vi "Fgen Channel UI.vi"() -> ()   [LabVIEW 2025, in "Fgen.lvlib" / "Fgen Channel.lvclass"]
doc: "Copyright 2017 National Instruments Corporation\n\nLicensed under the Apache License, Version 2.0 (the \"License\"); you may not use this file except in compliance with the License. You may obtain a copy of the License at http://www.apache.org/licenses/LICENSE-2.0\nUnless required by applicable law or agreed to in writing, software distributed under the License is distributed on an \"AS IS\" BASIS, WITHOUT WARRANTIES OR CONDITIONS OF ANY KIND, either express or implied. See the License for the specific language governing permissions and limitations under the License."
uses:
  Fgen Channel.lvclass
  Users/Public/Documents/Sandia National Labs/TSS Plugin/CEF.lvlibp/Node/NodeRef.ctl
  Users/Public/Documents/Sandia National Labs/TSS Plugin/CEF.lvlibp/Node/CEF_Node.lvclass
  Users/Public/Documents/Sandia National Labs/TSS Plugin/CEF.lvlibp/Node/mainQref.ctl
  Users/Public/Documents/Sandia National Labs/TSS Plugin/CEF.lvlibp/Node/UserEventRef.ctl
  Users/Public/Documents/Sandia National Labs/TSS Plugin/Abstract Engine.lvlibp/Plugin/Abstract/Channel configuration/Default Channel.ctl
  Fgen Channel configuration/Fgen Channel Setting.ctl
  Fgen Instrument/Fgen Instrument.lvclass
  Fgen Channel.lvclass/Fgen Channel.ctl
  Fgen Channel configuration/Fgen Channel configuration.lvclass/Fgen Channel configuration.ctl
  Fgen configuration/Fgen configuration.lvclass
  Fgen Channel configuration/Read Fgen Channel.vi
  Fgen Channel configuration/Write Fgen Channel.vi
  <vilib>/Utility/error.llb/Trim Whitespace One-Sided.vi
  Fgen Channel configuration/Fgen Channel configuration.lvclass
  Users/Public/Documents/Sandia National Labs/TSS Plugin/Abstract Engine.lvlibp/Plugin/Abstract/Channel configuration/Read Channel Setting.vi
  Users/Public/Documents/Sandia National Labs/TSS Plugin/CEF.lvlibp/Node/ReadParent.vi
  Users/Public/Documents/Sandia National Labs/TSS Plugin/Abstract Engine.lvlibp/Plugin/Abstract/Instrument configuration/Read Instrument Setting.vi
  Users/Public/Documents/Sandia National Labs/TSS Plugin/Abstract Engine.lvlibp/Plugin/Abstract/Channel configuration/Write Channel Setting.vi
  Users/Public/Documents/Sandia National Labs/TSS Plugin/CEF.lvlibp/serializable configuration/CEF_serializable configuration.lvclass
  Users/Public/Documents/Sandia National Labs/TSS Plugin/Abstract Engine.lvlibp/Plugin/Abstract/Channel configuration/Channel configuration.lvclass
panel:
  in  "Fgen Channel":cluster{"Default":T1, "Setting":T2}={"Default"={"Address"="None", "SW Alias"="Fgen Channel0", "Enabled"=TRUE, "Type"="Fgen Channel", "Description"="* Type = Channel Class"}, "Setting"={"Trgger Type"="Immediate", "Duty Cycle"=0.0, "Amplitude"=0.0, "Frequency"=0.0, "Output Shape"="Sine Wave", "Phase"=0.0}} {"Setting"."Duty Cycle" format="%#_6f"; "Setting"."Frequency" format="%#_6p"; "Setting"."Amplitude" format="%#_6f"}
  in  "user event":T3
  in  "main queue":T4
  in  "node ref":T5
  # "Standard only"
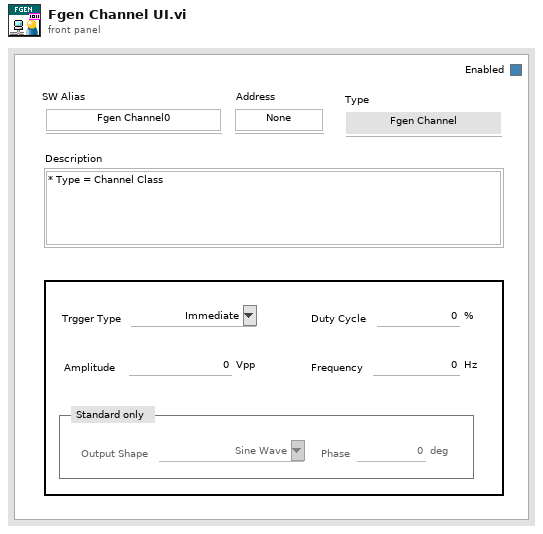
[diagram p1: front panel]
types:
  T1 = typedef "Abstract Engine.lvlibp/Channel configuration.lvclass/Default Channel.ctl" = cluster{"Address":string, "SW Alias":string, "Enabled":bool, "Type":string, "Description":string}
  T2 = typedef "Fgen.lvlib/Fgen Channel configuration.lvclass/Fgen Channel Setting.ctl" = cluster{"Trgger Type":string, "Duty Cycle":dbl, "Amplitude":dbl, "Frequency":dbl, "Output Shape":string, "Phase":dbl}
  T3 = typedef "CEF.lvlibp/CEF_Node.lvclass/UserEventRef.ctl" = refnum<user-event>
  T4 = typedef "CEF.lvlibp/CEF_Node.lvclass/mainQref.ctl" = refnum<queue>
  T5 = typedef "CEF.lvlibp/CEF_Node.lvclass/NodeRef.ctl" = refnum<data-value>
  T6 = typedef "Abstract Engine.lvlibp/Instrument configuration.lvclass/Default Instrument.ctl" = cluster{"Type":string, "Address":string, "SW Alias":string, "Description":string, "Enabled":bool}
  T7 = enum8{"Enabled", "Disabled", "Disabled and Grayed Out"}
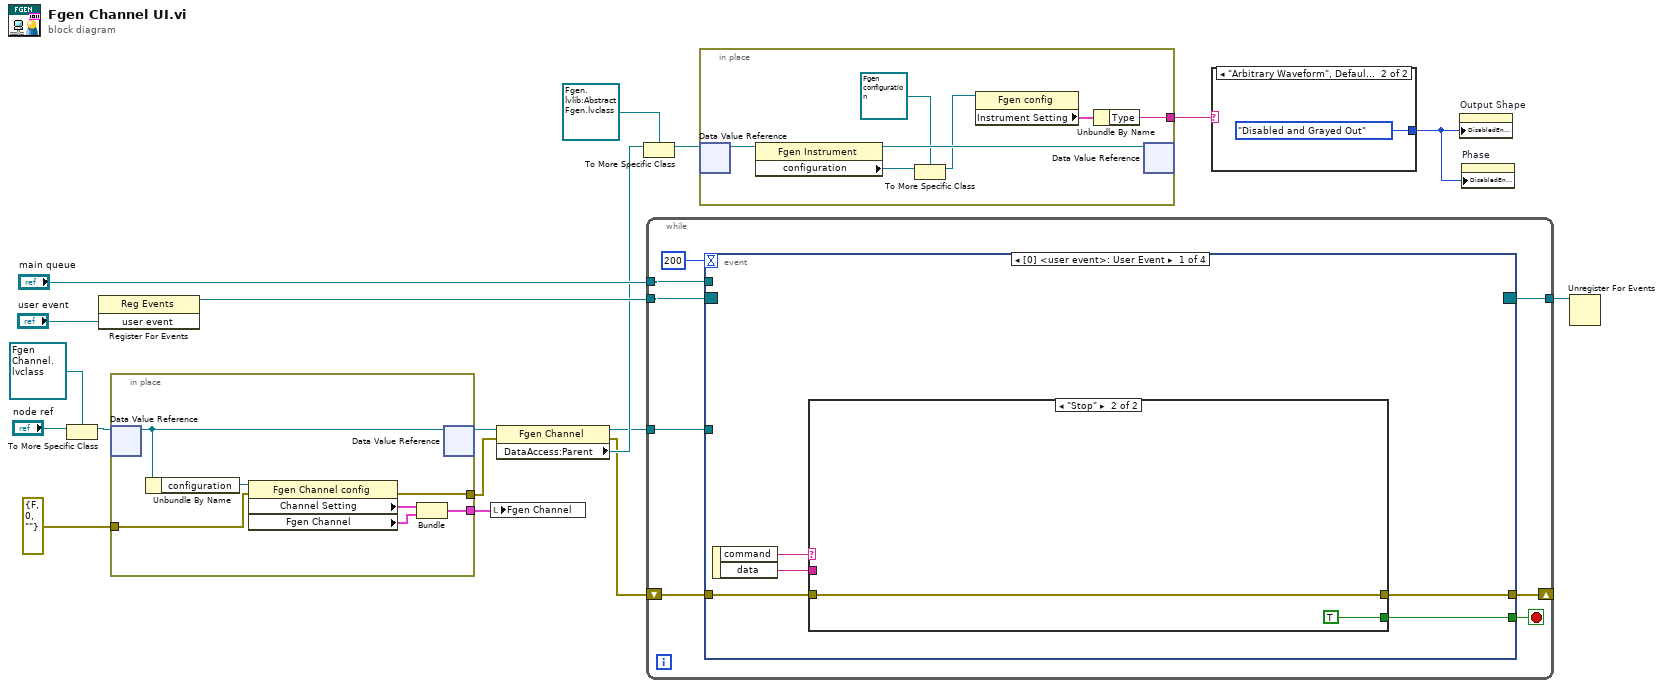
[diagram p0: block diagram]
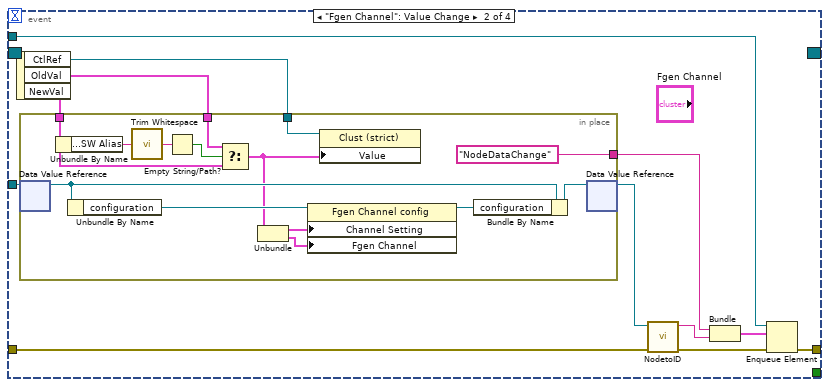
[diagram p3: hidden frame]
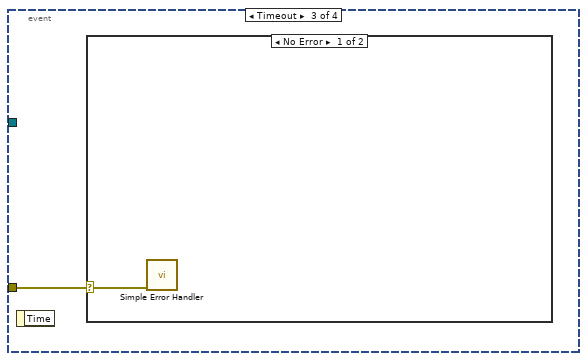
[diagram p4: hidden frame]
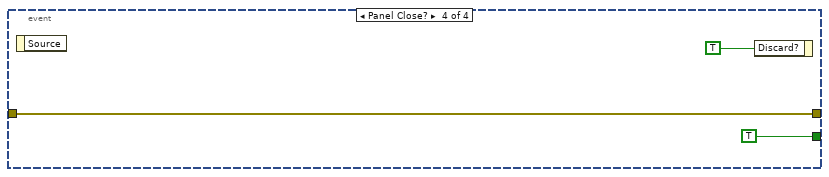
[diagram p6: hidden frame]
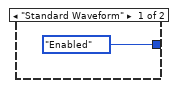
[diagram p7: hidden frame]
diagram:
  n1 = To More Specific Class(target class=refnum<data-value> refnum ("data value reference"), reference="node ref") -> (specific class reference=w8:refnum<data-value>)  [unwired: 1 in, 1 out]
  n2 = register-events("user event") -> (reference out=w17:refnum<event-registration>)  [unwired: 2 in, 1 out]
  n3 = in-place {
    in-place-border: [w21] -> w4
    in-place-border: errorcluster {"status"=FALSE, "code"=0, "source"=""} ("error out") -> [w20]
    in-place-border: [w19] -> w2
    # "Initialize the front panel controls when loaded"
    n4 = in-place-dvr #1(w8) -> (w24:refnum<class "Fgen Channel.lvclass">)  [unwired: 1 out]
    n5 = Unbundle By Name(w24) -> ("configuration"=w25:refnum<class "Fgen Channel configuration.lvclass">)
    n6 = property class="Fgen Channel config"(reference=w25, error in=w20) -> (error out=w19:errorcluster, "Channel Setting"=w23:T1, "Fgen Channel"=w22:T2)  [unwired: 1 out]
    n7 = Bundle("Channel Setting"=w23, "Fgen Channel"=w22) -> (w21:cluster{"Channel Setting":T1, "Fgen Channel":T2})  [unwired: 1 in]
    n8 = in-place-dvr #1(w24) -> (w7:refnum<data-value>)  [unwired: 1 out]
  }
  n9 = local write "Fgen Channel"(w4) -> ()
  n10 = property class="Fgen Channel"(reference=w7, error in=w2) -> (reference out=w10:refnum<data-value>, error out=w1:errorcluster, "DataAccess:Parent"=w11:refnum<data-value>)
  n11 = To More Specific Class(target class=refnum<data-value> refnum ("data value reference"), reference=w11) -> (specific class reference=w12:refnum<data-value>)  [unwired: 1 in, 1 out]
  n12 = while {
    tunnel: w10 -> [w33]
    tunnel: w17 -> [w32]
    tunnel: [w31] -> w16
    shift-right: [w28] -> _
    shift-left: w1 -> [w30]
    tunnel: "main queue" -> [w27]
    stop <- w29 stop-if-true
    n13 = event shown="[0] <user event>: User Event" {
      selector: w32 -> [_ _ _ _]
      dyn-events: [_ _ _ _] -> w31
      timeout: 200 -> [_ _ _ _]
      tunnel: w33 -> [_ w49 _ _]
      tunnel: [w34 w50 _ w70] -> w28
      tunnel: w30 -> [w35 w51 w68 w70]
      tunnel: [w38 _ _ TRUE] -> w29
      tunnel: w27 -> [_ w52 _ _]
      event User Event {
        n14 = event-data() -> ("command"=w36:string, "data"=w37:string)  [unwired: 1 in]
        n15 = case shown="\"Stop\"" w36 {
          tunnel: w37 -> [_ _]
          tunnel: [_ TRUE] -> w38
          tunnel: w35 -> [w39 w40]
          tunnel: [w39 w40] -> w34
          frame Default {
          }
          frame "Stop" {
          }
        }
      }
      event "Fgen Channel": Value Change {
        n16 = event-data() -> ("CtlRef"=w45:refnum<vi>, "OldVal"=w46:cluster{"Default":T1, "Setting":T2}, "NewVal"=w47:cluster{"Default":T1, "Setting":T2})  [unwired: 1 in]
        n17 = in-place {
          in-place-border: w47 -> [w60]
          in-place-border: w46 -> [w63]
          in-place-border: w45 -> [w62]
          in-place-border: ["NodeDataChange" ("Message Name")] -> w43
          n18 = in-place-dvr #2(w49) -> (w67:refnum<class "Fgen Channel.lvclass">)  [unwired: 1 out]
          n19 = Unbundle By Name(w60) -> ("Default.SW Alias"=w61:string)
          n20 = Unbundle By Name(w67) -> ("configuration"=w65:refnum<class "Fgen Channel configuration.lvclass">)
          n21 = call <vilib>:"Trim Whitespace.vi"("string"=w61) -> ("trimmed string"=w58:string)  [unwired: 1 in]
          n22 = Empty String/Path?(string/path=w58) -> (empty?=w59:bool)
          n23 = Select(t=w63, s=w59, f=w60) -> (s? t:f=w57:cluster{"Default":T1, "Setting":T2})
          n24 = Unbundle(w57) -> ("Default"=w54:T1, "Setting"=w56:T2)
          n25 = property class="Fgen Channel config"(reference=w65, "Channel Setting"=w54, "Fgen Channel"=w56) -> (reference out=w64:refnum<class "Fgen Channel configuration.lvclass">)  [unwired: 1 in, 1 out]
          n26 = property class="Clust (strict)"(reference=w62, "Value"=w57) -> ()  [unwired: 1 in, 2 out]
          n27 = Bundle By Name(cluster=w67, "configuration"=w64) -> (w66:refnum<class "Fgen Channel.lvclass">)
          n28 = in-place-dvr #2(w66) -> (w48:refnum<data-value>)  [unwired: 1 out]
        }
        n29 = call "NodetoID.vi"("error in"=w51, "node ref"=w48) -> ("error out"=w53:errorcluster, "ID"=w44:string)  [unwired: 8 in]
        n30 = Bundle("Message Name"=w43, "ID"=w44) -> (w42:cluster{"Message Name":string, "ID":string})  [unwired: 1 in]
        n31 = Enqueue Element(queue=w52, element=w42, error in (no error)=w53) -> (error out=w50:errorcluster)  [unwired: 1 in, 2 out]
      }
      event Timeout {
        n32 = event-data() -> ()  [unwired: 1 in, 1 out]
        n33 = case shown="No Error" w68 {
          selector: w68 -> [w69 _]
          frame No Error {
            n34 = call <vilib>:"Simple Error Handler.vi"("error in (no error)"=w69) -> ()  [unwired: 4 in, 5 out]
          }
          frame Error {
          }
        }
      }
      event Panel Close? {
        n35 = event-data() -> ()  [unwired: 1 in, 1 out]
        n36 = event-data("Discard?"=TRUE) -> ()  [unwired: 1 in, 1 out]
      }
    }
  }
  n37 = in-place {
    in-place-border: [w79] -> w9
    # "Initialize the front panel controls when loaded"
    n38 = in-place-dvr #3(w12) -> (w78:refnum<class "Fgen Instrument.lvclass">)  [unwired: 1 out]
    n39 = property class="Fgen Instrument"(reference=w78) -> (reference out=w77:refnum<class "Fgen Instrument.lvclass">, "configuration"=w76:refnum<class "CEF_serializable configuration.lvclass">)  [unwired: 1 in, 1 out]
    n40 = To More Specific Class(target class=refnum<class "Fgen configuration.lvclass"> refnum ("Fgen.lvlib:Fgen configuration.lvclass"), reference=w76) -> (specific class reference=w74:refnum<class "Fgen configuration.lvclass">)  [unwired: 1 in, 1 out]
    n41 = property class="Fgen config"(reference=w74) -> ("Instrument Setting"=w73:T6)  [unwired: 1 in, 2 out]
    n42 = Unbundle By Name(w73) -> ("Type"=w79:string)
    n43 = in-place-dvr #3(w77) -> ()  [unwired: 2 out]
  }
  n44 = case shown="\"Arbitrary Waveform\", Default" w9 {
    tunnel: [T7."Enabled" ("Disabled") T7."Disabled and Grayed Out" ("Disabled")] -> w6
    frame "Standard Waveform" {
    }
    frame "Arbitrary Waveform", Default {
    }
  }
  n45 = property on="Output Shape" class="CmbBox"("DisabledEnum"=w6) -> ()  [unwired: 2 in, 2 out]
  n46 = property on="Phase" class="DigNum (strict)"("DisabledEnum"=w6) -> ()  [unwired: 2 in, 2 out]
  n47 = Unregister For Events(event registration refnum=w16) -> ()  [unwired: 1 in, 1 out]
